vi "moveAndRetrieveToCheckKingToKing.vi"(1 "j2":i32, 2 "i2":i32, 3 "j1":i32, 4 "i1":i32) -> (0 "isKingToKing":bool)   [LabVIEW 2024]
uses:
  globalVar.vi
panel:
  out "eg2":i32
  out "eg1":i32
  out "ep2":i32
  out "ep1":i32
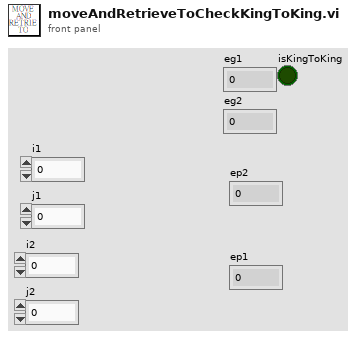
[diagram p1: front panel]
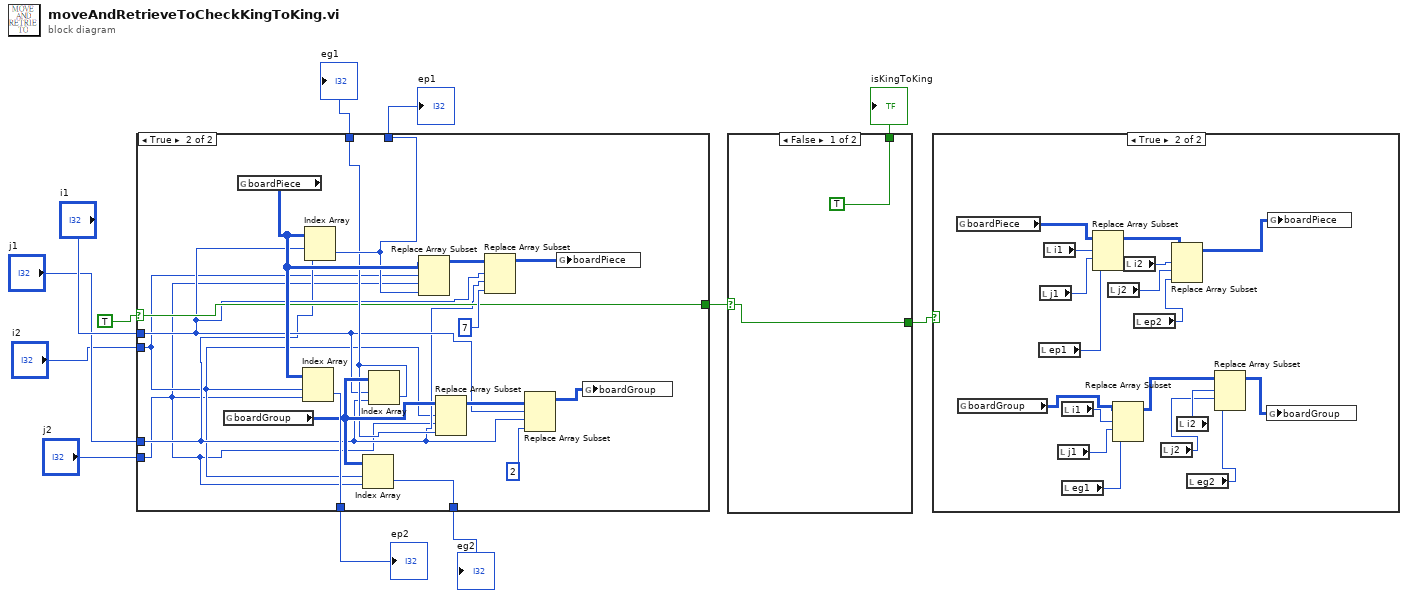
[diagram p0: block diagram]
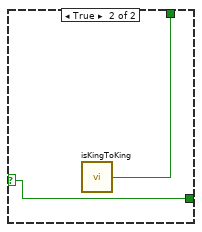
[diagram p3: hidden frame]
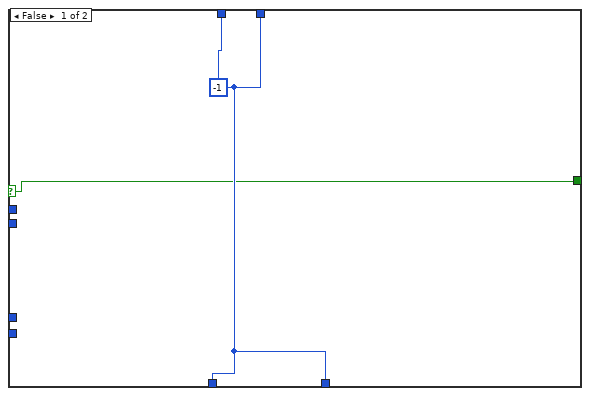
[diagram p4: hidden frame]
diagram:
  n1 = case shown="True" TRUE {
    selector: TRUE -> [w13 w19]
    tunnel: [w14 w30] -> w11
    tunnel: [w14 w29] -> w10
    tunnel: [w14 w23] -> w9
    tunnel: [w14 w26] -> w8
    tunnel: [w13 w19] -> w7
    tunnel: "i1" -> [_ w18]
    tunnel: "j1" -> [_ w17]
    tunnel: "i2" -> [_ w16]
    tunnel: "j2" -> [_ w15]
    frame False {
      w14 = -1 ("Numeric")
    }
    frame True {
      n2 = global read "globalVar.vi" "boardGroup"() -> (w25:i32[][])
      n3 = global read "globalVar.vi" "boardPiece"() -> (w31:i32[][])
      n4 = Index Array(array=w31, index (row)=w16, index (col)=w15) -> (element=w30:i32)
      n5 = Index Array(array=w31, index (row)=w18, index (col)=w17) -> (element=w29:i32)
      n6 = Index Array(array=w25, index (row)=w16, index (col)=w15) -> (element=w26:i32)
      n7 = Index Array(array=w25, index (row)=w18, index (col)=w17) -> (element=w23:i32)
      n8 = Replace Array Subset(array=w31, new element=w29, index (row)=w16, index (col)=w15) -> (w28:i32[][])
      n9 = Replace Array Subset(array=w25, new element=w23, index (row)=w16, index (col)=w15) -> (w24:i32[][])
      n10 = Replace Array Subset(array=w28, new element=7 ("new element/subarray"), index (row)=w18, index (col)=w17) -> (w20:i32[][])
      n11 = Replace Array Subset(array=w24, new element=2 ("new element/subarray"), index (row)=w18, index (col)=w17) -> (w21:i32[][])
      n12 = global write "globalVar.vi" "boardPiece"(w20) -> ()
      n13 = global write "globalVar.vi" "boardGroup"(w21) -> ()
    }
  }
  "ep2" <- w11
  "ep1" <- w10
  "eg1" <- w9
  "eg2" <- w8
  n14 = case shown="False" w7 {
    selector: w7 -> [w32 w34]
    tunnel: [TRUE ("isKingToKing") w35] -> w6
    tunnel: [w32 w34] -> w1
    frame False {
    }
    frame True {
      n15 = call "isKingToKing.vi"() -> ("isKingToKing"=w35:bool)
    }
  }
  "isKingToKing" <- w6
  n16 = case shown="True" w1 {
    frame False {
    }
    frame True {
      n17 = global read "globalVar.vi" "boardPiece"() -> (w53:i32[][])
      n18 = global read "globalVar.vi" "boardGroup"() -> (w44:i32[][])
      n19 = local read "ep1"() -> (w52:i32)
      n20 = local read "j1"() -> (w48:i32)
      n21 = local read "i1"() -> (w49:i32)
      n22 = local read "j1"() -> (w42:i32)
      n23 = local read "i1"() -> (w43:i32)
      n24 = local read "eg1"() -> (w41:i32)
      n25 = Replace Array Subset(array=w53, new element=w52, index (row)=w49, index (col)=w48) -> (w51:i32[][])
      n26 = local read "j2"() -> (w46:i32)
      n27 = Replace Array Subset(array=w44, new element=w41, index (row)=w43, index (col)=w42) -> (w37:i32[][])
      n28 = local read "i2"() -> (w47:i32)
      n29 = local read "ep2"() -> (w45:i32)
      n30 = local read "j2"() -> (w39:i32)
      n31 = Replace Array Subset(array=w51, new element=w45, index (row)=w47, index (col)=w46) -> (w50:i32[][])
      n32 = local read "i2"() -> (w40:i32)
      n33 = local read "eg2"() -> (w38:i32)
      n34 = Replace Array Subset(array=w37, new element=w38, index (row)=w40, index (col)=w39) -> (w36:i32[][])
      n35 = global write "globalVar.vi" "boardGroup"(w36) -> ()
      n36 = global write "globalVar.vi" "boardPiece"(w50) -> ()
    }
  }
